vi "浊度电极校准.vi"() -> ()   [LabVIEW 2016, in "斯坦道多参数.lvlib"]
uses:
  <vilib>/Analysis/NI_AALBase.lvlib
  <vilib>/Plasmionique/MB Master/MB_Master_Serial/MB_Master_Serial.lvclass
  C:/Program Files (x86)/National Instruments/LabVIEW 2016/vi.lib/Plasmionique/MB Master/MB_Master/MB_Master.lvclass
panel:
  out "mean":dbl caption="均值" format="%0.2f"
  out "standard deviation":dbl caption="标准差" format="%0.2f"
  out "变异系数":dbl
  out "测量值":dbl
  out "提示":string
  in  "第二点通过校正":bool
  in  "第一点通过校正":bool
  in  "第二点校正":bool
  in  "第一点校正":bool
  out "标液2":dbl
  out "标液1":dbl
  out "原始读取值":dbl caption="信号值"
  out "偏移值补偿":dbl
  out "电极斜率":dbl
  out "电极零点":dbl
  # "浊度电极设定"
  # "NTU"
  # "NTU"
  # "%"
  # "NTU"
  # "NTU"
  # "电极校正"
  # "标准液值:"
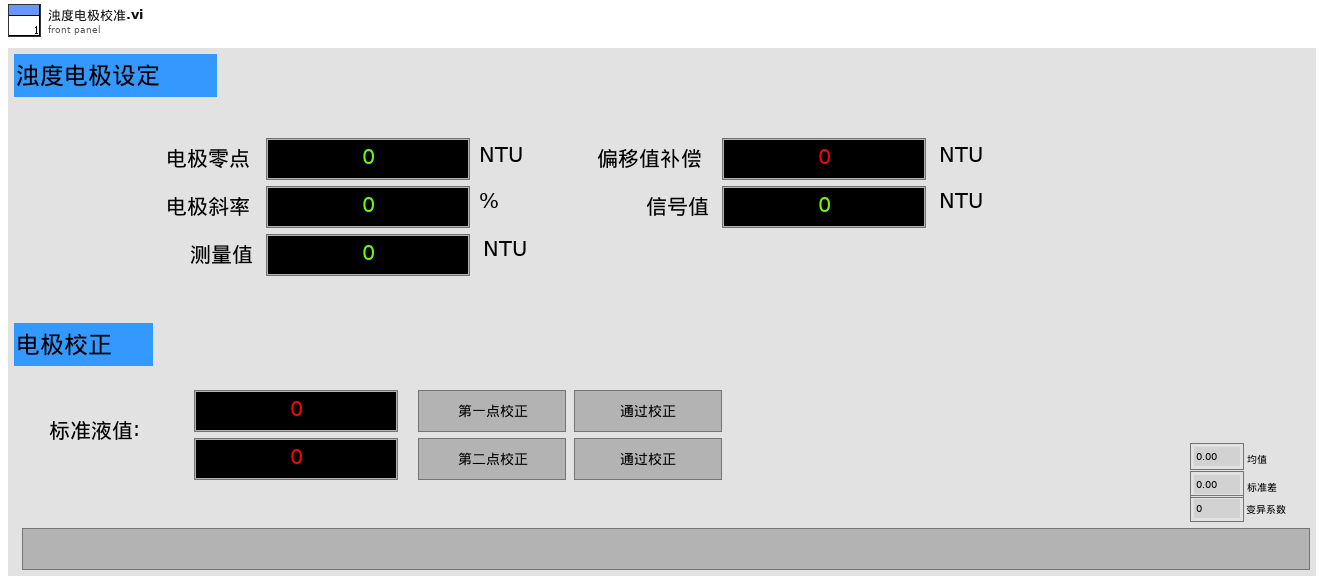
[diagram p1: front panel]
types:
  T1 = typedef "斯坦道多参数.lvlib/校准步骤.ctl" = enum16{"待机", "放置第一点标液", "第一点校准启动", "第一点校准写入", "第一点校准失败", "放置第二点标液", "第二点校准启动", "第二点校准写入", "第二点校准失败", "校准结果写入", "校准结束"}
  T2 = cluster{"电极状态标志":u16, "电极型号标志":u16, "浊度测量值":sgl, "温度测量值":sgl, "浊度信号值":sgl, "浊度偏移修正值":sgl, "温度偏移修正值":sgl, "手动温度补偿值":sgl, "浊度电极零点":sgl, "浊度电极斜率":sgl, "第1点标准值记录":sgl, "第1点信号值记录":sgl, "第1点温度值记录":sgl, "第2点标准值记录":sgl, "第2点信号值记录":sgl, "第2点温度值记录":sgl, "命令滤波设定":u16, "温度模式":enum16{"ATC", "MTC"}, "生产批次":u16, "电极序号":u16, "串口地址":u16, "串口波特率":enum16{"9600", "19200", "115200"}, "串口校验位":enum16{"NONE", "ODD", "EVEN"}, "串口停止位":enum16{"1bit", "2bit"}, "第一点标准值":sgl, "第二点标准值":sgl}
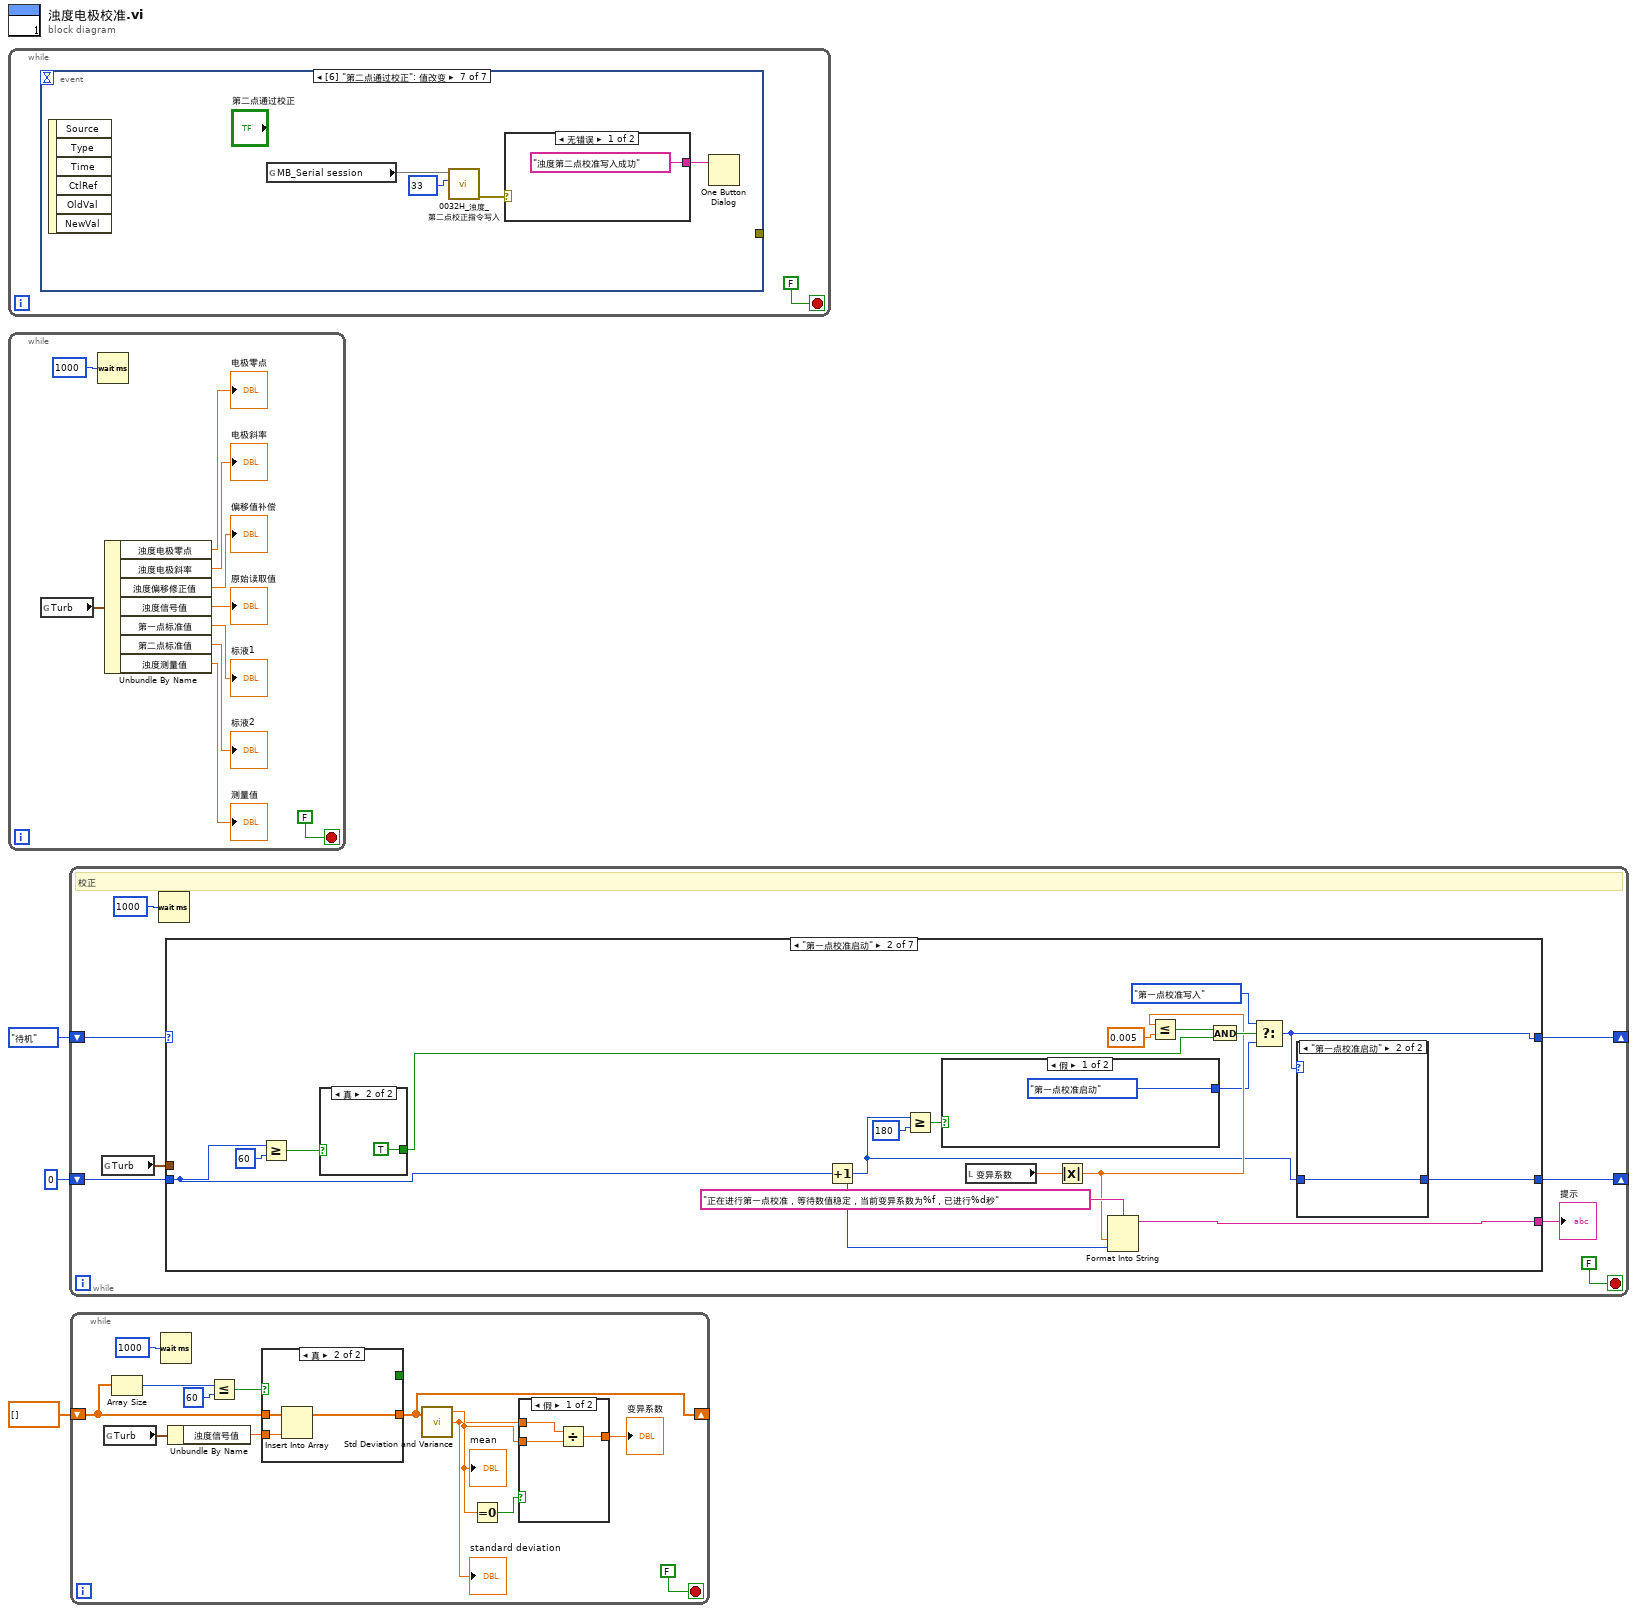
[diagram p0: block diagram]
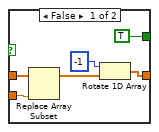
[diagram p3: hidden frame]
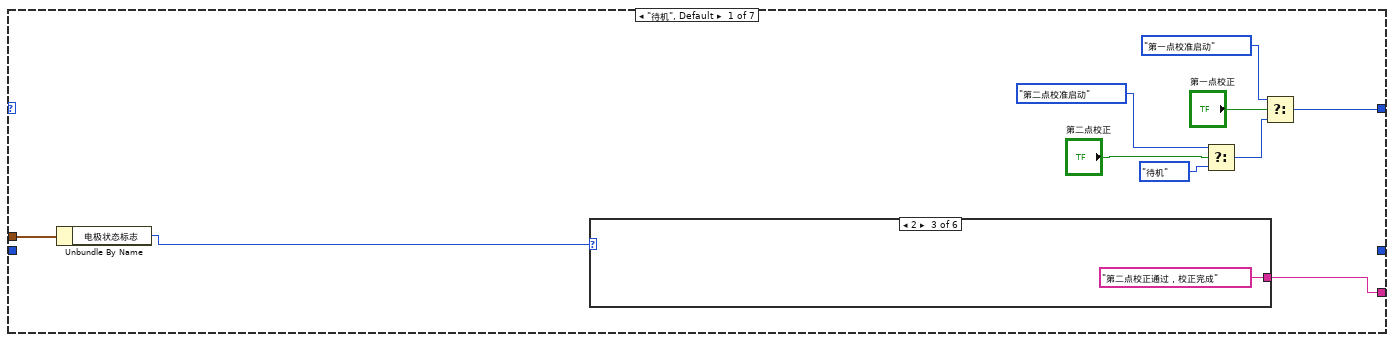
[diagram p4: hidden frame]
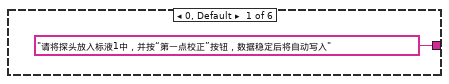
[diagram p5: hidden frame]
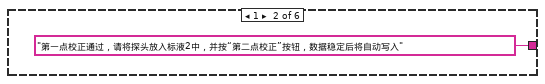
[diagram p6: hidden frame]
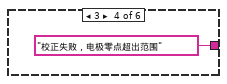
[diagram p7: hidden frame]
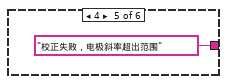
[diagram p8: hidden frame]
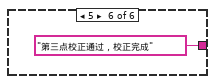
[diagram p9: hidden frame]
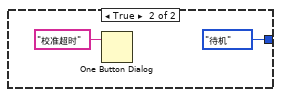
[diagram p11: hidden frame]
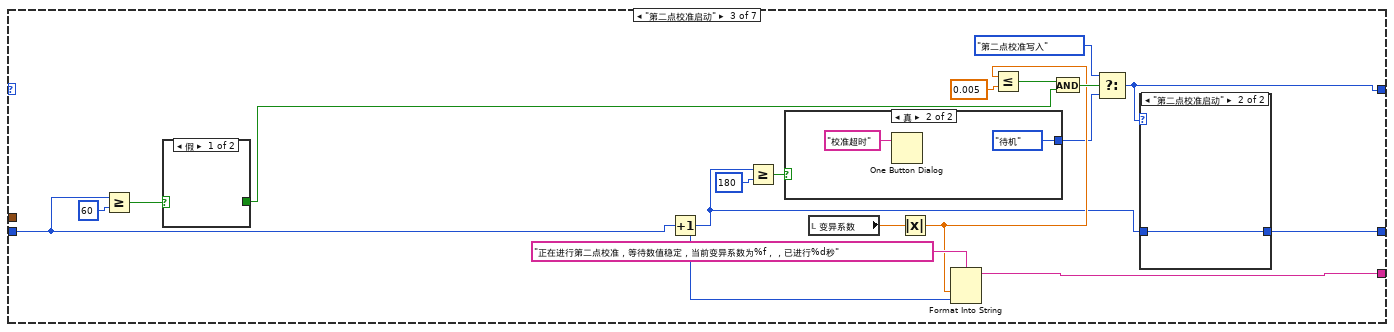
[diagram p13: hidden frame]
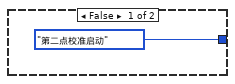
[diagram p15: hidden frame]
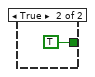
[diagram p16: hidden frame]
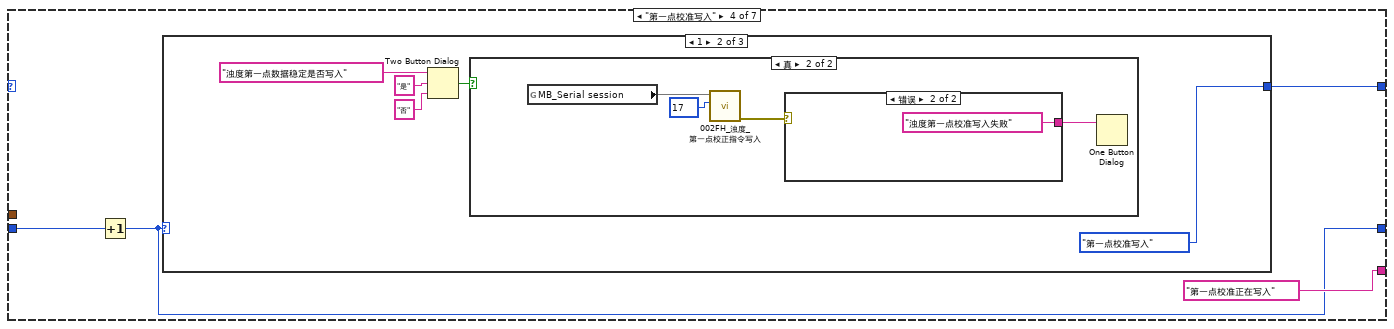
[diagram p17: hidden frame]
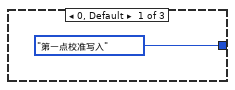
[diagram p18: hidden frame]
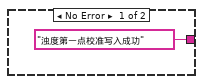
[diagram p20: hidden frame]
diagram:
  n1 = while {
    stop <- FALSE stop-if-true
    n2 = event shown="[6] \"第二点通过校正\": 值改变" {
      selector: _ -> [_ _ _ _ _ _ _]
      dyn-events: _ -> [_ _ _ _ _ _ _]
      timeout: _ -> [_ _ _ _ _ _ _]
      tunnel: [_ _ w9 w12 w16 _ _] -> _
      event Timeout {
        n3 = event-data() -> ()  [unwired: 1 in, 3 out]
      }
      event "偏移值补偿", "标液1", "标液2": Mouse Down {
        n4 = event-data() -> ("CtlRef"=w5:refnum<vi>)  [unwired: 1 in, 7 out]
        n5 = property class="DigNum (严格)"(reference=w5) -> (reference out=w6:refnum<vi>, "Value"=w7:dbl)  [unwired: 1 in, 1 out]
        n6 = call "数字键盘.vi"("OldNumber"=w7) -> ("NewNumber"=w8:sgl)
        n7 = property class="DigNum (严格)"(reference=w6, "Val(Sgnl)"=w8) -> ()  [unwired: 1 in, 2 out]
      }
      event "偏移值补偿": Value Change {
        n8 = event-data() -> ("NewVal"=w10:dbl)  [unwired: 1 in, 5 out]
        n9 = global read "国弘过程全局变量.vi" "MB_Serial session"() -> (w11)
        n10 = call "000CH_浊度_浊度偏移修正值写入.vi"("数值"=w10, "MB_Serial session in"=w11) -> ("error out"=w9:errorcluster)  [unwired: 8 in, 1 out]
      }
      event "标液1": Value Change {
        n11 = event-data() -> ("NewVal"=w14:dbl)  [unwired: 1 in, 5 out]
        n12 = global read "国弘过程全局变量.vi" "MB_Serial session"() -> (w13)
        n13 = call "0030H_浊度_第一点标准值写入.vi"("数值"=w14, "MB_Serial session in"=w13) -> ("error out"=w12:errorcluster)  [unwired: 8 in, 1 out]
      }
      event "标液2": Value Change {
        n14 = event-data() -> ("NewVal"=w15:dbl)  [unwired: 1 in, 5 out]
        n15 = global read "国弘过程全局变量.vi" "MB_Serial session"() -> (w17)
        n16 = call "0033H_浊度_第二点标准值写入.vi"("数值"=w15, "MB_Serial session in"=w17) -> ("error out"=w16:errorcluster)  [unwired: 8 in, 1 out]
      }
      event "第一点通过校正": Value Change {
        n17 = event-data() -> ()  [unwired: 1 in, 6 out]
        n18 = global read "国弘过程全局变量.vi" "MB_Serial session"() -> (w21)
        n19 = call "002FH_浊度_第一点校正指令写入.vi"("数值"=u16 17, "MB_Serial session in"=w21) -> ("error out"=w18:errorcluster)  [unwired: 8 in, 1 out]
        n20 = case shown="错误" w18 {
          tunnel: ["浊度第一点校准写入成功" ("消息") "浊度第一点校准写入失败" ("消息")] -> w19
          frame No Error {
          }
          frame Error {
          }
        }
        n21 = One Button Dialog(message=w19) -> ()  [unwired: 1 in, 1 out]
      }
      event "第二点通过校正": Value Change {
        n22 = event-data() -> ()  [unwired: 1 in, 6 out]
        n23 = global read "国弘过程全局变量.vi" "MB_Serial session"() -> (w26)
        n24 = call "0032H_浊度_第二点校正指令写入.vi"("数值"=u16 33, "MB_Serial session in"=w26) -> ("error out"=w24:errorcluster)  [unwired: 8 in, 1 out]
        n25 = case shown="无错误" w24 {
          tunnel: ["浊度第二点校准写入成功" ("消息") "浊度第二点校准写入失败" ("消息")] -> w25
          frame No Error {
          }
          frame Error {
          }
        }
        n26 = One Button Dialog(message=w25) -> ()  [unwired: 1 in, 1 out]
      }
    }
  }
  n27 = while {
    stop <- FALSE stop-if-true
    n28 = global read "国弘过程全局变量.vi" "Turb"() -> (w37:T2)
    n29 = Wait (ms)(milliseconds to wait=u32 1000 ("等待时间（毫秒）")) -> ()  [unwired: 1 out]
    n30 = Unbundle By Name(w37) -> ("浊度电极零点"=→"电极零点":sgl, "浊度电极斜率"=→"电极斜率":sgl, "浊度偏移修正值"=→"偏移值补偿":sgl, "浊度信号值"=→"原始读取值":sgl, "第一点标准值"=→"标液1":sgl, "第二点标准值"=→"标液2":sgl, "浊度测量值"=→"测量值":sgl)
  }
  n31 = while "While循环" {
    shift-right: [w46] -> _
    shift-left: 校准步骤."待机" ("枚举") -> [w47]
    shift-right: [w41] -> _
    shift-left: 0 -> [w42]
    stop <- FALSE stop-if-true
    # "校正"
    n32 = global read "国弘过程全局变量.vi" "Turb"() -> (w44:T2)
    n33 = Wait (ms)(milliseconds to wait=u32 1000 ("等待时间（毫秒）")) -> ()  [unwired: 1 out]
    n34 = case shown="\"第一点校准启动\"" w47 {
      tunnel: [w56 w68 w91 w110 w127 校准步骤."待机" ("枚举") 校准步骤."待机" ("枚举")] -> w46
      tunnel: [w54 w78 w96 "第一点校准正在写入" ("提示") "第二点校准正在写入" ("提示") "第一点校准失败" ("提示") "第二点校准失败" ("提示")] -> w40
      tunnel: w44 -> [w53 _ _ _ _ _ _]
      tunnel: w42 -> [_ w65 w88 w112 w129 w145 w150]
      tunnel: [_ w66 w89 w111 w128 w144 w149] -> w41
      frame "待机", Default {
        n35 = Unbundle By Name(w53) -> ("电极状态标志"=w55:u16)
        n36 = case shown="2" w55 {
          tunnel: ["请将探头放入标液1中，并按“第一点校正”按钮，数据稳定后将自动写入" ("提示") "第一点校正通过，请将探头放入标液2中，并按“第二点校正”按钮，数据稳定后将自动写入" ("提示") "第二点校正通过，校正完成" ("提示") "校正失败，电极零点超出范围" ("提示") "校正失败，电极斜率超出范围" ("提示") "第三点校正通过，校正完成" ("提示")] -> w54
          frame 0, Default {
          }
          frame 1 {
          }
          frame 2 {
          }
          frame 3 {
          }
          frame 4 {
          }
          frame 5 {
          }
        }
        n37 = Select(t=校准步骤."第二点校准启动" ("枚举"), s="第二点校正", f=校准步骤."待机" ("枚举")) -> (s? t:f=w50:T1)
        n38 = Select(t=校准步骤."第一点校准启动" ("枚举"), s="第一点校正", f=w50) -> (s? t:f=w56:T1)
      }
      frame "第一点校准启动" {
        n39 = Greater Or Equal?(x=w65, y=60) -> (x >= y?=w80:bool)
        n40 = case shown="真" w80 {
          tunnel: [_ TRUE] -> w75
          frame False {
          }
          frame True {
          }
        }
        n41 = Increment(x=w65) -> (x+1=w67:i32)
        n42 = Greater Or Equal?(x=w67, y=180) -> (x >= y?=w70:bool)
        n43 = case shown="假" w70 {
          tunnel: [校准步骤."第一点校准启动" ("枚举") 校准步骤."待机" ("枚举")] -> w69
          frame False {
          }
          frame True {
            n44 = One Button Dialog(message="校准超时" ("消息")) -> ()  [unwired: 1 in, 1 out]
          }
        }
        n45 = local read "变异系数"() -> (w64:dbl)
        n46 = Absolute Value(x=w64) -> (abs(x)=w72:dbl)
        n47 = Format Into String(format string="正在进行第一点校准，等待数值稳定，当前变异系数为%f，已进行%d秒" ("格式字符串"), w72, w67) -> (resulting string=w78:string)  [unwired: 2 in, 1 out]
        n48 = Less Or Equal?(x=w72, y=0.005) -> (x <= y?=w74:bool)
        n49 = And(x=w74, y=w75) -> (x .and. y?=w73:bool)
        n50 = Select(t=校准步骤."第一点校准写入" ("枚举"), s=w73, f=w69) -> (s? t:f=w68:T1)
        n51 = case shown="\"第一点校准启动\"" w68 {
          tunnel: w67 -> [_ w82]
          tunnel: [_ w82] -> w66
          frame "待机", Default {
          }
          frame "第一点校准启动" {
          }
        }
      }
      frame "第二点校准启动" {
        n52 = Greater Or Equal?(x=w88, y=60) -> (x >= y?=w103:bool)
        n53 = case shown="假" w103 {
          tunnel: [_ TRUE] -> w99
          frame False {
          }
          frame True {
          }
        }
        n54 = Increment(x=w88) -> (x+1=w90:i32)
        n55 = Greater Or Equal?(x=w90, y=180) -> (x >= y?=w93:bool)
        n56 = case shown="真" w93 {
          tunnel: [校准步骤."第二点校准启动" ("枚举") 校准步骤."待机" ("枚举")] -> w92
          frame False {
          }
          frame True {
            n57 = One Button Dialog(message="校准超时" ("消息")) -> ()  [unwired: 1 in, 1 out]
          }
        }
        n58 = local read "变异系数"() -> (w87:dbl)
        n59 = Absolute Value(x=w87) -> (abs(x)=w95:dbl)
        n60 = Format Into String(format string="正在进行第二点校准，等待数值稳定，当前变异系数为%f，，已进行%d秒" ("格式字符串"), w95, w90) -> (resulting string=w96:string)  [unwired: 2 in, 1 out]
        n61 = Less Or Equal?(x=w95, y=0.005) -> (x <= y?=w98:bool)
        n62 = And(x=w98, y=w99) -> (x .and. y?=w97:bool)
        n63 = Select(t=校准步骤."第二点校准写入" ("枚举"), s=w97, f=w92) -> (s? t:f=w91:T1)
        n64 = case shown="\"第二点校准启动\"" w91 {
          tunnel: w90 -> [_ w105]
          tunnel: [_ w105] -> w89
          frame "待机", Default {
          }
          frame "第二点校准启动" {
          }
        }
      }
      frame "第一点校准写入" {
        n65 = Increment(x=w112) -> (x+1=w111:i32)
        n66 = case shown="1" w111 {
          tunnel: [校准步骤."第一点校准写入" ("枚举") 校准步骤."第一点校准写入" ("枚举") 校准步骤."待机" ("枚举")] -> w110
          frame 0, Default {
          }
          frame 1 {
            n67 = Two Button Dialog(message="浊度第一点数据稳定是否写入" ("消息"), 1:"否" ("F按钮名称（“取消”）"), 2:"是" ("T按钮名称（“确定”）")) -> (T button?=w115:bool)
            n68 = case shown="真" w115 {
              frame False {
              }
              frame True {
                n69 = global read "国弘过程全局变量.vi" "MB_Serial session"() -> (w123)
                n70 = call "002FH_浊度_第一点校正指令写入.vi"("数值"=u16 17, "MB_Serial session in"=w123) -> ("error out"=w120:errorcluster)  [unwired: 8 in, 1 out]
                n71 = case shown="错误" w120 {
                  tunnel: ["浊度第一点校准写入成功" ("消息") "浊度第一点校准写入失败" ("消息")] -> w121
                  frame No Error {
                  }
                  frame Error {
                  }
                }
                n72 = One Button Dialog(message=w121) -> ()  [unwired: 1 in, 1 out]
              }
            }
          }
          frame 2 {
          }
        }
      }
      frame "第二点校准写入" {
        n73 = Increment(x=w129) -> (x+1=w128:i32)
        n74 = case shown="1" w128 {
          tunnel: [校准步骤."第二点校准写入" ("枚举") 校准步骤."第二点校准写入" ("枚举") 校准步骤."待机" ("枚举")] -> w127
          frame 0, Default {
          }
          frame 1 {
            n75 = Two Button Dialog(message="浊度第二点数据稳定是否写入" ("消息"), 1:"否" ("F按钮名称（“取消”）"), 2:"是" ("T按钮名称（“确定”）")) -> (T button?=w132:bool)
            n76 = case shown="真" w132 {
              frame False {
              }
              frame True {
                n77 = global read "国弘过程全局变量.vi" "MB_Serial session"() -> (w139)
                n78 = call "0032H_浊度_第二点校正指令写入.vi"("数值"=u16 33, "MB_Serial session in"=w139) -> ("error out"=w137:errorcluster)  [unwired: 8 in, 1 out]
                n79 = case shown="错误" w137 {
                  tunnel: ["浊度第二点校准写入成功" ("消息") "浊度第二点校准写入失败" ("消息")] -> w138
                  frame No Error {
                  }
                  frame Error {
                  }
                }
                n80 = One Button Dialog(message=w138) -> ()  [unwired: 1 in, 1 out]
              }
            }
          }
          frame 2 {
          }
        }
      }
      frame "第一点校准失败" {
        n81 = Two Button Dialog(message="第一点校准失败是否重新校准" ("消息")) -> ()  [unwired: 2 in, 1 out]
        n82 = Increment(x=w145) -> (x+1=w144:i32)
      }
      frame "第二点校准失败" {
        n83 = Increment(x=w150) -> (x+1=w149:i32)
      }
    }
    "提示" <- w40
  }
  n84 = while {
    shift-right: [w158] -> _
    shift-left: sgl[] [] -> [w161]
    stop <- FALSE stop-if-true
    n85 = global read "国弘过程全局变量.vi" "Turb"() -> (w153:T2)
    n86 = Array Size(array=w161) -> (size(s)=w163:i32)
    n87 = Wait (ms)(milliseconds to wait=u32 1000 ("等待时间（毫秒）")) -> ()  [unwired: 1 out]
    n88 = Unbundle By Name(w153) -> ("浊度信号值"=w160:sgl)
    n89 = Less Or Equal?(x=w163, y=60) -> (x <= y?=w162:bool)
    n90 = case shown="真" w162 {
      tunnel: w161 -> [w174 w177]
      tunnel: w160 -> [w172 w176]
      tunnel: [w170 w175] -> w158
      tunnel: [TRUE _] -> _
      frame False {
        n91 = Replace Array Subset(array=w174, new element=w172) -> (w173:sgl[])  [unwired: 1 in]
        n92 = Rotate 1D Array(1:w173, 2:-1 ("n")) -> (0:w170:sgl[])
      }
      frame True {
        n93 = Insert Into Array(array=w177, new element=w176) -> (w175:sgl[])  [unwired: 1 in]
      }
    }
    n94 = call <vilib>:"Std Deviation and Variance.vi"("X"=w158) -> ("mean"=w157:dbl, "standard deviation"=w156:dbl)  [unwired: 1 in, 1 out]
    "mean" <- w157
    "standard deviation" <- w156
    n95 = Equal To 0?(x=w157) -> (x = 0?=w159:bool)
    n96 = case shown="假" w159 {
      tunnel: w156 -> [w168 _]
      tunnel: [w167 _] -> w155
      tunnel: w157 -> [w166 _]
      frame False {
        n97 = Divide(x=w168, y=w166) -> (x/y=w167:dbl)
      }
      frame True {
      }
    }
    "变异系数" <- w155
  }
